vi "Analog.vi"(8 "error in (no error)":errorcluster, 10 "K":sgl=3.32, 11 "Analog In in":T2) -> (0 "error out":errorcluster, 2 "Volage":dbl(knob) scale=0.0..15.0, 3 "Analog In out":T1)   [LabVIEW 2020]
uses:
  <vilib>/High Genius/HG_WSI_Tookit/Dependencies/Library/Analog In/Analog In.lvclass
  C:/Program Files (x86)/National Instruments/LabVIEW 2020/vi.lib/High Genius/HG_WSI_Tookit/Dependencies/Library/HG_LIB/HG_LIB.lvclass
  <vilib>/High Genius/HG_WSI_Tookit/Dependencies/Library/HG_LIB/HG_LIB.lvclass/HG_LIB.ctl
  <vilib>/High Genius/HG_WSI_Tookit/Dependencies/Library/HG_LIB/HG_LIB.lvclass
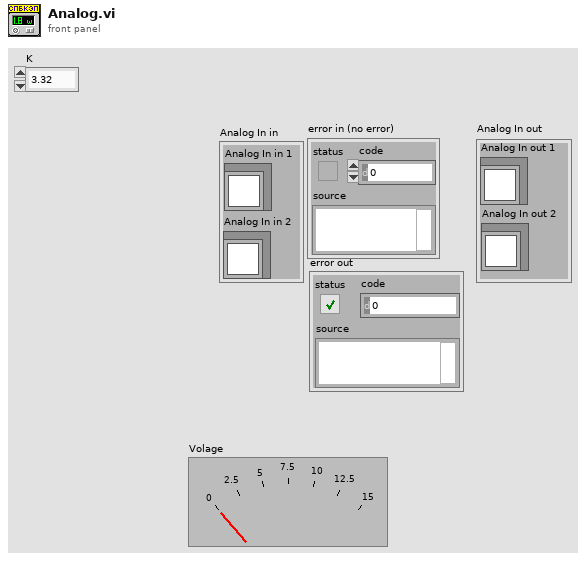
[diagram p1: front panel]
types:
  T1 = cluster{"Analog In out 1":refnum<class "Analog In.lvclass">, "Analog In out 2":refnum<class "Analog In.lvclass">}
  T2 = cluster{"Analog In in 1":refnum<class "Analog In.lvclass">, "Analog In in 2":refnum<class "Analog In.lvclass">}
  T3 = cluster{"data":cluster{"ai22":sgl, "ai23":sgl, "ai24":sgl, "ai25":sgl, "pulse12":i32, "pulse13":i32, "pwm14":i32, "pwm15":i32, "pwm16":i32, "do17":bool, "do18":bool, "do19":bool, "do20":bool, "do21":bool, "di11":bool, "di9":bool, "motor0":u8, "motor1":u8, "motor2":u8, "motor3":u8, "dir00":u8, "dir01":u8, "dir02":u8, "dir03":u8, "dir10":u8, "dir11":u8, "dir12":u8, "dir13":u8, "limit0":bool, "limit1":bool, "limit2":bool, "limit3":bool, "limit4":bool, "limit5":bool, "limit6":bool, "limit7":bool, "lsb0H":u8, "lsb1H":u8, "lsb2H":u8, "lsb3H":u8, "lsb0L":u8, "lsb1L":u8, "lsb2L":u8, "lsb3L":u8, "enc0_counters":u32, "enc1_counters":u32, "enc2_counters":u32, "enc3_counters":u32, "counter10":u32, "counter8":u32, "reset_enc0":bool, "reset_enc1":bool, "reset_enc2":bool, "reset_enc3":bool, "pitch":sgl, "roll":sgl, "yaw":sgl, "zero_yaw":bool}}
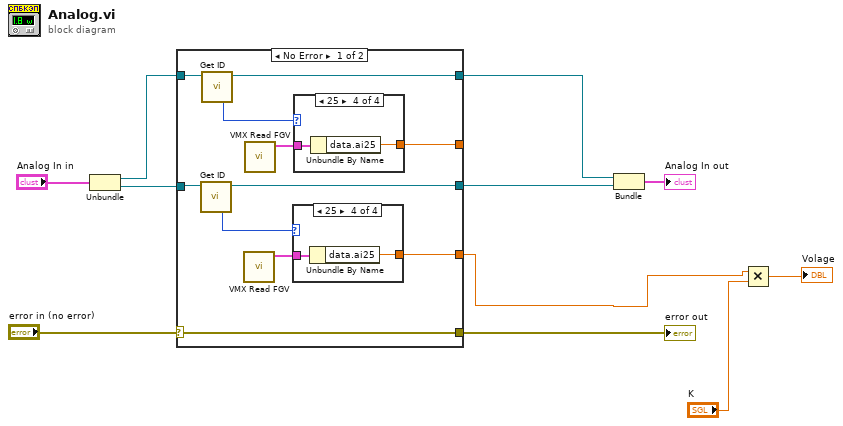
[diagram p0: block diagram]
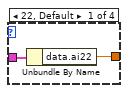
[diagram p2: hidden frame]
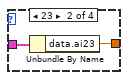
[diagram p3: hidden frame]
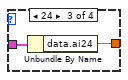
[diagram p4: hidden frame]
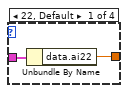
[diagram p5: hidden frame]
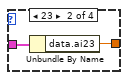
[diagram p6: hidden frame]
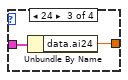
[diagram p7: hidden frame]
diagram:
  n1 = Unbundle("Analog In in") -> ("Analog In in 1"=w4:refnum<class "Analog In.lvclass">, "Analog In in 2"=w5:refnum<class "Analog In.lvclass">)
  n2 = case shown="No Error" "error in (no error)" {
    selector: "error in (no error)" -> [w18 w41]
    tunnel: [w18 w41] -> w8
    tunnel: [w22 w40] -> w6
    tunnel: w4 -> [w17 w40]
    tunnel: [w19 _] -> _
    tunnel: w5 -> [w14 w39]
    tunnel: [w13 _] -> w3
    tunnel: [w12 w39] -> w7
    frame No Error {
      n3 = call <vilib>:"Get ID.vi"("HG_LIB in"=w14) -> ("ID"=w16:u32, "HG_LIB out"=w12:refnum<class "Analog In.lvclass">)  [unwired: 9 in]
      n4 = call <vilib>:"Get ID.vi"("HG_LIB in"=w17) -> ("ID"=w20:u32, "HG_LIB out"=w22:refnum<class "Analog In.lvclass">)  [unwired: 9 in]
      n5 = call <vilib>:"VMX Read FGV.vi"() -> ("Read Data"=w15:T3)  [unwired: 10 in, 1 out]
      n6 = call <vilib>:"VMX Read FGV.vi"() -> ("Read Data"=w21:T3)  [unwired: 10 in, 1 out]
      n7 = case shown="25" w16 {
        tunnel: w15 -> [w24 w26 w27 w30]
        tunnel: [w23 w25 w28 w29] -> w13
        frame 22, Default {
          n8 = Unbundle By Name(w24) -> ("data.ai22"=w23:sgl)
        }
        frame 23 {
          n9 = Unbundle By Name(w26) -> ("data.ai23"=w25:sgl)
        }
        frame 24 {
          n10 = Unbundle By Name(w27) -> ("data.ai24"=w28:sgl)
        }
        frame 25 {
          n11 = Unbundle By Name(w30) -> ("data.ai25"=w29:sgl)
        }
      }
      n12 = case shown="25" w20 {
        tunnel: w21 -> [w32 w34 w35 w38]
        tunnel: [w31 w33 w36 w37] -> w19
        frame 22, Default {
          n13 = Unbundle By Name(w32) -> ("data.ai22"=w31:sgl)
        }
        frame 23 {
          n14 = Unbundle By Name(w34) -> ("data.ai23"=w33:sgl)
        }
        frame 24 {
          n15 = Unbundle By Name(w35) -> ("data.ai24"=w36:sgl)
        }
        frame 25 {
          n16 = Unbundle By Name(w38) -> ("data.ai25"=w37:sgl)
        }
      }
    }
    frame Error {
    }
  }
  "error out" <- w8
  n17 = Bundle("Analog In in 1"=w6, "Analog In in 2"=w7) -> (→"Analog In out":T2)  [unwired: 1 in]
  n18 = Multiply(x=w3, y="K") -> (x*y=→"Volage":sgl)
